vi "GetPathOfDotGitFolder.vi"() -> (2 "Number of nested git modules":i32, 3 ".git folder paths":path[](array[path]))   [LabVIEW 2018, in "feGEM DataPacker.lvlib"]
uses:
  feGEM DataPacker.lvlib
  <userlib>/_RADE/MTA-lib/file/file.llb/Valid Path - Traditional__ogtk.vi
  <userlib>/_RADE/MTA-lib/file/file.llb/Build Path - Traditional__ogtk.vi
panel:
  out ".git folder found":bool
  out "Valid Path":bool
  out "error out":errorcluster
  out "VI Path":path
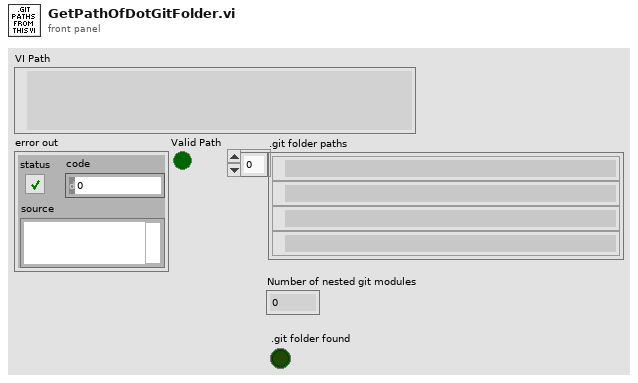
[diagram p1: front panel]
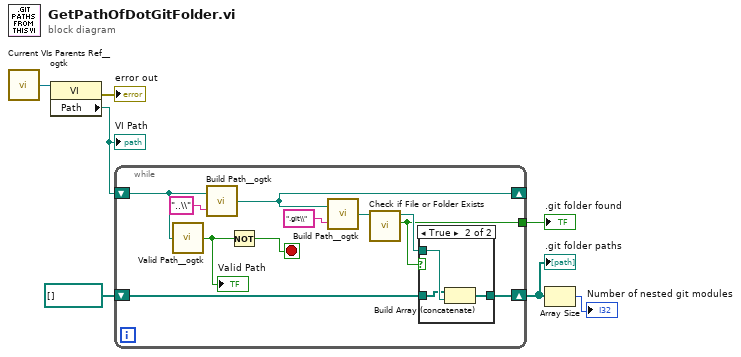
[diagram p0: block diagram]
diagram:
  n1 = call <userlib>:"Current VIs Parents Ref__ogtk.vi"() -> ("Calling VI's reference"=w7:refnum<vi>)  [unwired: 2 in]
  n2 = property class="VI"(reference=w7) -> (error out=→"error out":errorcluster, "Path"=w5:path)  [unwired: 1 in, 1 out]
  "VI Path" <- w5
  n3 = while {
    shift-right: [w16] -> _
    shift-left: w5 -> [w13]
    tunnel: [w9] -> w4
    shift-right: [w11] -> w3
    shift-left: path[] [] -> [w10]
    stop <- w8 stop-if-true
    n4 = call-poly <userlib>:"Valid Path__ogtk.vi"("path"=w13) -> ("valid"=w18:bool)
    "Valid Path" <- w18
    n5 = call-poly <userlib>:"Build Path__ogtk.vi"("name or relative path"="..\\", "base path"=w13) -> ("appended path"=w16:path)
    n6 = Not(x=w18) -> (.not. x?=w8:bool)
    n7 = call-poly <userlib>:"Build Path__ogtk.vi"("name or relative path"=".git\\", "base path"=w16) -> ("appended path"=w14:path)
    n8 = call <vilib>:"Check if File or Folder Exists.vi"("path"=w14) -> ("file or folder exists?"=w9:bool, "dup path"=w12:path)  [unwired: 8 in, 1 out]
    n9 = case shown="True" w9 {
      tunnel: w12 -> [_ w22]
      tunnel: [w19 w21] -> w11
      tunnel: w10 -> [w19 w20]
      frame False {
      }
      frame True {
        n10 = Build Array (concatenate)(w20, w22) -> (w21:path[])
      }
    }
  }
  ".git folder found" <- w4
  ".git folder paths" <- w3
  n11 = Array Size(array=w3) -> (size(s)=→"Number of nested git modules":i32)
